vi "LCR_PlotNamer.vi"(5 "Y-Axis":T4, 7 "X-Axis":T4, 9 "Param":enum16{"S11", "S21", "S12", "S22"}(ring), 10 "Parameter Plots":refnum<vi>, 11 "T/B Ref In":refnum<vi>) -> ()   [LabVIEW 2021]
uses:
  Plotting-Axis.ctl
  Data_Cluster.ctl
  Measurement_Cluster.ctl
  Mode_Enum.ctl
panel:
  out "Data_Out":T1={"Value"=0.0, "GUI Data Cluster"={"S11"=FALSE, "S21"=FALSE, "S12"=FALSE, "S22"=FALSE, "S11Meas"=enum."Log-magnitude (dB)", "S21Meas"=enum."Log-magnitude (dB)", "S12Meas"=enum."Log-magnitude (dB)", "S22Meas"=enum."Log-magnitude (dB)"}, "Timing"={"Last Operation"=0.0, "Stop @ T/B"=FALSE, "Last Temp"=0.0, "Last Mag"=0.0, "Ramp Param"={"End T (K)"=0.0, "Delta T (K)"=0.0, "End B (T)"=0.0, "Delta B (T)"=0.0}, "LastOp?"=FALSE}, "Measurements"=[], "Hardware"={"VNA TCP Con"=refnum, "VNA TCP Port"=5025, "Global T VAR"="", "Global B VAR"=""}, "Operation"={"Operation Mode"=enum."Logging", "Log Folder"=path "", "Measure Mode"=enum."Deltat"}}
  in  "Data_IN":T1={"Value"=0.0, "GUI Data Cluster"={"S11"=FALSE, "S21"=FALSE, "S12"=FALSE, "S22"=FALSE, "S11Meas"=enum."Log-magnitude (dB)", "S21Meas"=enum."Log-magnitude (dB)", "S12Meas"=enum."Log-magnitude (dB)", "S22Meas"=enum."Log-magnitude (dB)"}, "Timing"={"Last Operation"=0.0, "Stop @ T/B"=FALSE, "Last Temp"=0.0, "Last Mag"=0.0, "Ramp Param"={"End T (K)"=0.0, "Delta T (K)"=0.0, "End B (T)"=0.0, "Delta B (T)"=0.0}, "LastOp?"=FALSE}, "Measurements"=[], "Hardware"={"VNA TCP Con"=refnum, "VNA TCP Port"=5025, "Global T VAR"="", "Global B VAR"=""}, "Operation"={"Operation Mode"=enum."Logging", "Log Folder"=path "", "Measure Mode"=enum."Deltat"}}
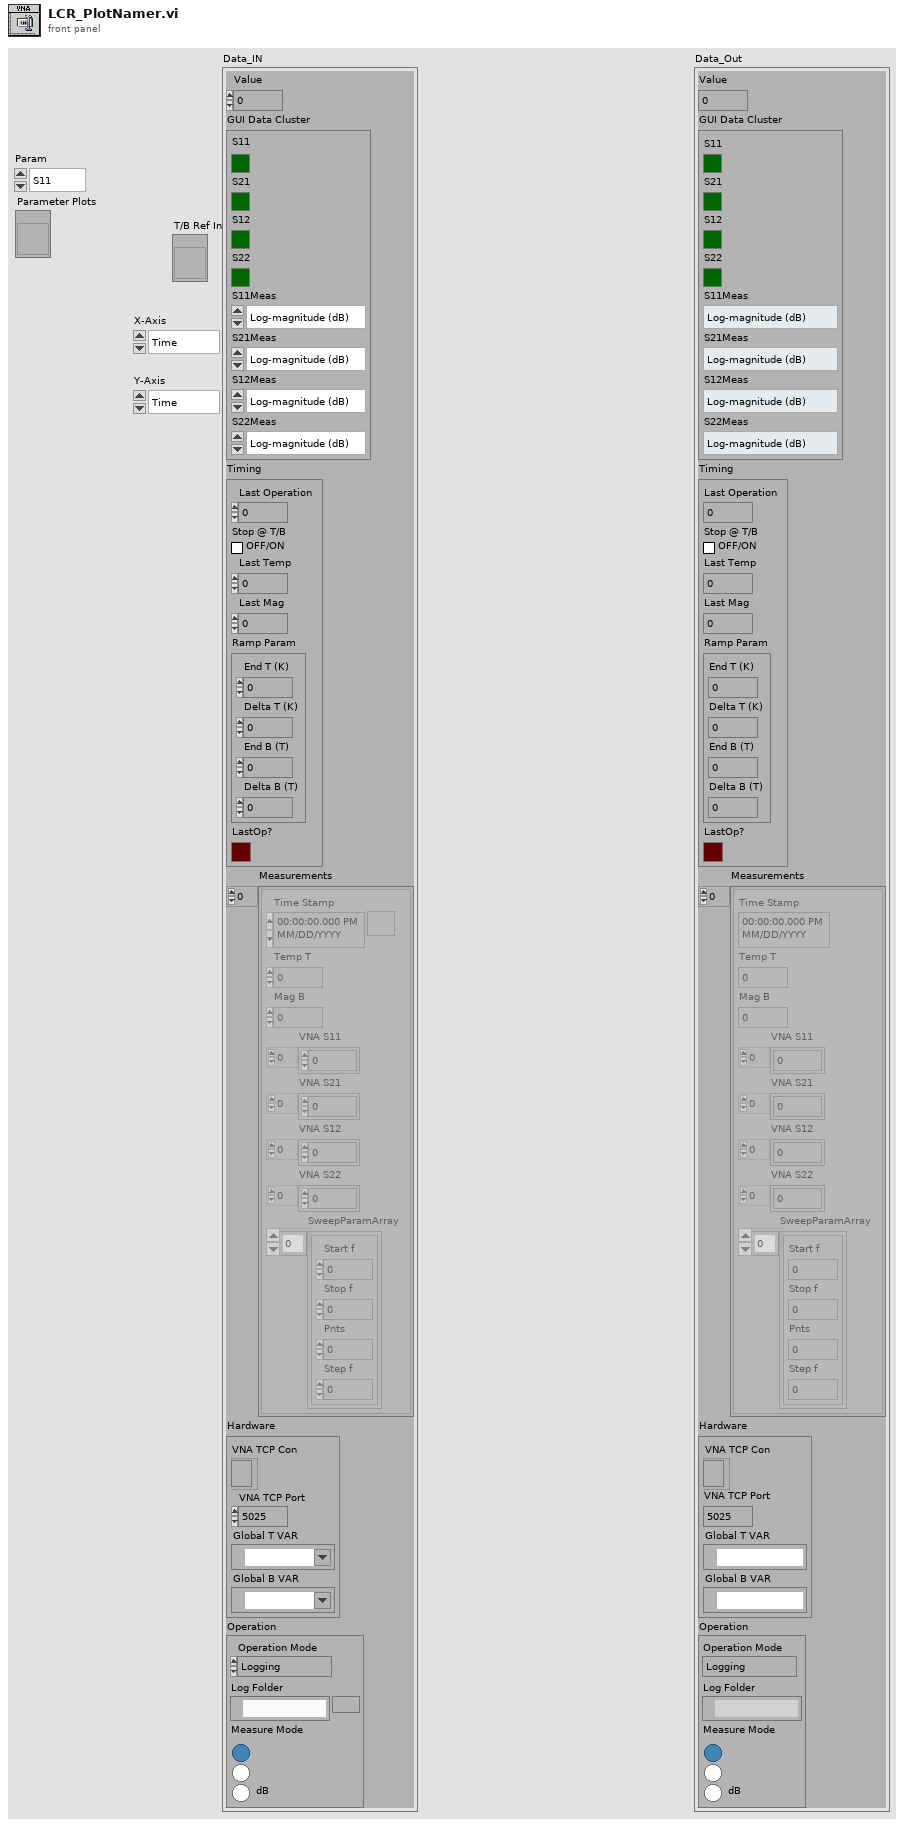
[diagram p1: front panel]
types:
  T1 = typedef "Data_Cluster.ctl" = cluster{"Value":dbl, "GUI Data Cluster":cluster{"S11":bool, "S21":bool, "S12":bool, "S22":bool, "S11Meas":enum16{"Log-magnitude (dB)", "Linear magnitude", "Phase (deg)", "Time Domain", "Real", "Imaginary", "Group Delay", "Polarlinear"}, "S21Meas":enum16{"Log-magnitude (dB)", "Linear magnitude", "Phase (deg)", "Time Domain", "Real", "Imaginary", "Group Delay", "Polarlinear"}, "S12Meas":enum16{"Log-magnitude (dB)", "Linear magnitude", "Phase (deg)", "Time Domain", "Real", "Imaginary", "Group Delay", "Polarlinear"}, "S22Meas":enum16{"Log-magnitude (dB)", "Linear magnitude", "Phase (deg)", "Time Domain", "Real", "Imaginary", "Group Delay", "Polarlinear"}}, "Timing":cluster{"Last Operation":dbl, "Stop @ T/B":bool, "Last Temp":dbl, "Last Mag":dbl, "Ramp Param":cluster{"End T (K)":dbl, "Delta T (K)":dbl, "End B (T)":dbl, "Delta B (T)":dbl}, "LastOp?":bool}, "Measurements":T2[], "Hardware":cluster{"VNA TCP Con":refnum<k5>, "VNA TCP Port":i32, "Global T VAR":refnum<k21>, "Global B VAR":refnum<k21>}, "Operation":cluster{"Operation Mode":T3, "Log Folder":path, "Measure Mode":enum32{"Deltat", "DeltaT", "dB"}}}
  T2 = typedef "Measurement_Cluster.ctl" = cluster{"Time Stamp":timestamp, "Temp T":dbl, "Mag B":dbl, "VNA S11":dbl[], "VNA S21":dbl[], "VNA S12":dbl[], "VNA S22":dbl[], "SweepParamArray":cluster{"Start f":dbl, "Stop f":dbl, "Pnts":i32, "Step f":dbl}[]}
  T3 = typedef "Mode_Enum.ctl" = enum16{"Logging", "Idle-Off", "Idle"}
  T4 = typedef "Plotting-Axis.ctl" = enum16{"Time", "Temperature", "Magnetic Field"}
  T5 = enum16{"Log-magnitude (dB)", "Linear magnitude", "Phase (deg)", "Time Domain", "Real", "Imaginary", "Group Delay", "Polarlinear"}
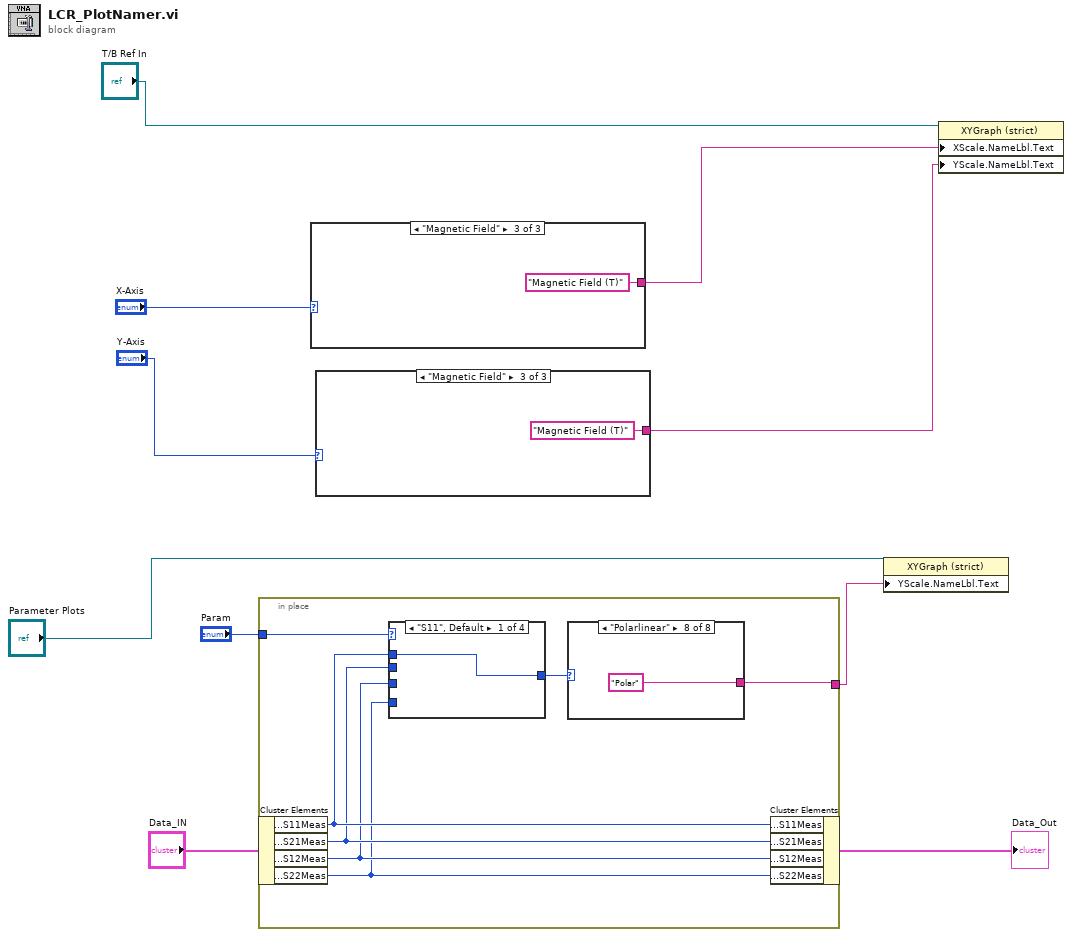
[diagram p0: block diagram]
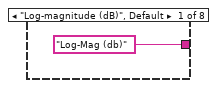
[diagram p2: hidden frame]
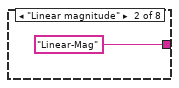
[diagram p3: hidden frame]
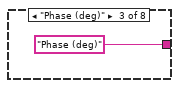
[diagram p4: hidden frame]
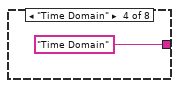
[diagram p5: hidden frame]
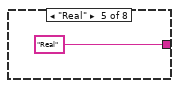
[diagram p6: hidden frame]
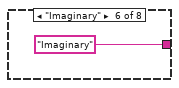
[diagram p7: hidden frame]
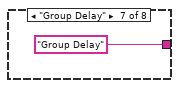
[diagram p8: hidden frame]
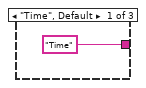
[diagram p12: hidden frame]
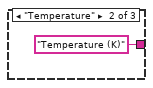
[diagram p13: hidden frame]
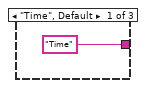
[diagram p14: hidden frame]
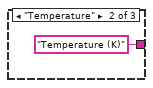
[diagram p15: hidden frame]
diagram:
  n1 = in-place {
    in-place-border: "Param" -> [w17]
    in-place-border: [w14] -> w2
    n2 = in-place-cluster #1("Data_IN") -> ("GUI Data Cluster.S11Meas"=w16:T5, "GUI Data Cluster.S21Meas"=w13:T5, "GUI Data Cluster.S12Meas"=w12:T5, "GUI Data Cluster.S22Meas"=w11:T5)
    n3 = case shown="\"S11\", Default" w17 {
      tunnel: w16 -> [w26 _ _ _]
      tunnel: [w26 w27 w28 w29] -> w15
      tunnel: w13 -> [_ w27 _ _]
      tunnel: w12 -> [_ _ w28 _]
      tunnel: w11 -> [_ _ _ w29]
      frame "S11", Default {
      }
      frame "S21" {
      }
      frame "S12" {
      }
      frame "S22" {
      }
    }
    n4 = case shown="\"Polarlinear\"" w15 {
      tunnel: ["Log-Mag (db)" "Linear-Mag" "Phase (deg)" "Time Domain" "Real" "Imaginary" "Group Delay" "Polar"] -> w14
      frame "Log-magnitude (dB)", Default {
      }
      frame "Linear magnitude" {
      }
      frame "Phase (deg)" {
      }
      frame "Time Domain" {
      }
      frame "Real" {
      }
      frame "Imaginary" {
      }
      frame "Group Delay" {
      }
      frame "Polarlinear" {
      }
    }
    n5 = in-place-cluster #1("GUI Data Cluster.S11Meas"=w16, "GUI Data Cluster.S21Meas"=w13, "GUI Data Cluster.S12Meas"=w12, "GUI Data Cluster.S22Meas"=w11) -> (→"Data_Out":T1)
  }
  n6 = case shown="\"Magnetic Field\"" "X-Axis" {
    tunnel: ["Time" "Temperature (K)" ("Caption.Text") "Magnetic Field (T)" ("Caption.Text")] -> w7
    frame "Time", Default {
    }
    frame "Temperature" {
    }
    frame "Magnetic Field" {
    }
  }
  n7 = case shown="\"Magnetic Field\"" "Y-Axis" {
    tunnel: ["Time" "Temperature (K)" ("Caption.Text") "Magnetic Field (T)" ("Caption.Text")] -> w6
    frame "Time", Default {
    }
    frame "Temperature" {
    }
    frame "Magnetic Field" {
    }
  }
  n8 = property class="XYGraph (strict)"(reference="Parameter Plots", "YScale.NameLbl.Text"=w2) -> ()  [unwired: 1 in, 2 out]
  n9 = property class="XYGraph (strict)"(reference="T/B Ref In", "XScale.NameLbl.Text"=w7, "YScale.NameLbl.Text"=w6) -> ()  [unwired: 1 in, 2 out]
